vi "Display QDList Function.vi"(8 "error in (no error)":errorcluster, 9 "QDFunction Acronym(\"\")":string, 10 "QDFunction Name(\"\")":string, 11 "NormalQDFunc in":refnum<class "QDDialogList.lvclass">) -> (0 "error out":errorcluster, 2 "Content For Display":string, 3 "NormalQDFunc out":refnum<class "QDDialogList.lvclass">)   [LabVIEW 2015, in "QDDialogList.lvclass"]
uses:
  <vilib>/LazyBootMenu/QDSearchList/QDDialogList.lvclass
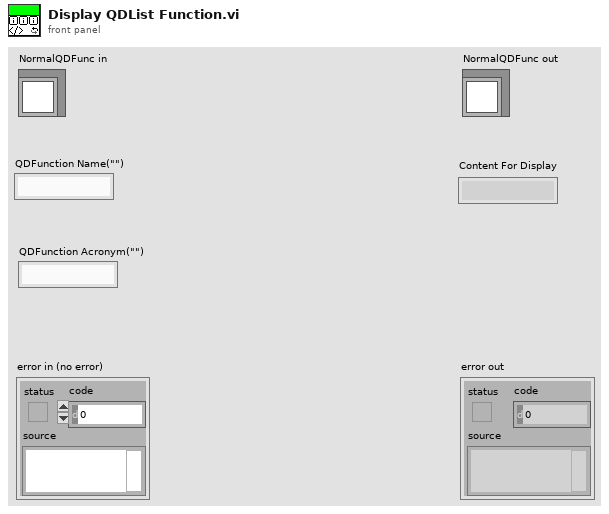
[diagram p1: front panel]
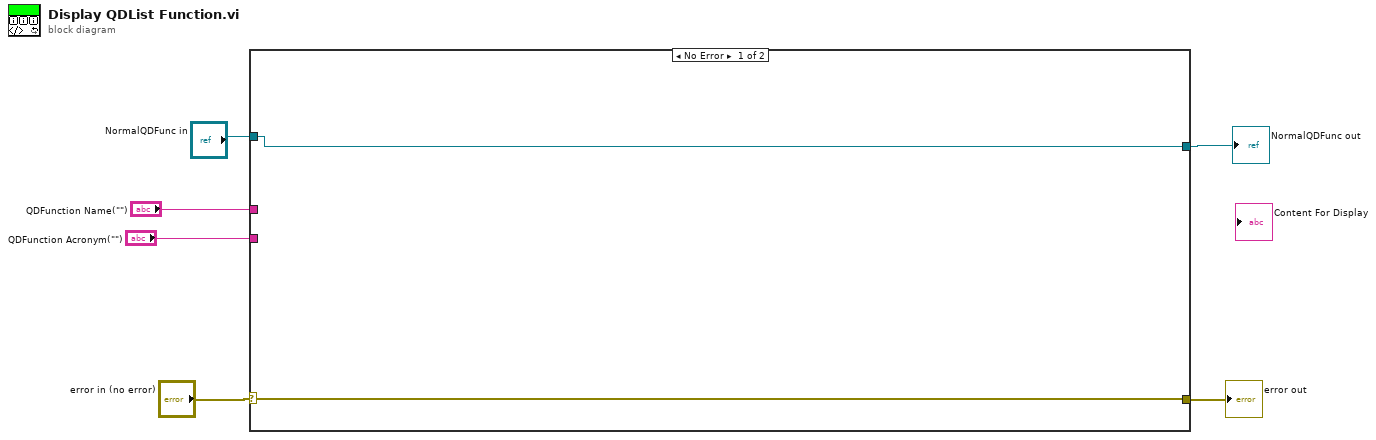
[diagram p0: block diagram]
diagram:
  n1 = case shown="No Error" "error in (no error)" {
    selector: "error in (no error)" -> [w8 w10]
    tunnel: "NormalQDFunc in" -> [w7 w9]
    tunnel: [w8 w10] -> w4
    tunnel: [w7 w9] -> w3
    tunnel: "QDFunction Name(\"\")" -> [_ _]
    tunnel: "QDFunction Acronym(\"\")" -> [_ _]
    frame No Error {
    }
    frame Error {
    }
  }
  "error out" <- w4
  "NormalQDFunc out" <- w3
